vi "HFRR ADV v01.vi"() -> ()   [LabVIEW 2025] (continued)
    "Single" <- "Single - Graph"
  }
  n1798 = disable-structure shown="Disabled" {
    disable-tunnel: [w1922 _] -> w48
    disable-tunnel: _ -> [w1921 _]
    frame Disabled {
      n1799 = while {
        tunnel: w1921 -> [_]
        tunnel: [w1923] -> w1922
        tunnel: [w1924] -> _
        i -> [w1924]
        stop <- w1923 stop-if-true
        w1940 = u16 10 items=["1.0"=10, "1.5"=15, "2.0"=20] ("stop bits (10: 1 bit)")
        n1800 = Wait (ms)(milliseconds to wait=u32 10) -> ()  [unwired: 1 out]
        n1801 = call-poly "VISA Configure Serial Port"("VISA resource name"=refnum<visa-resource-name> "ASRL1::INSTR" ("COM PORT"), "timeout (10sec)"=u32 10, "baud rate (9600)"=u32 57600, "data bits (8)"=u16 8, "stop bits (10: 1 bit)"=w1940) -> ("VISA resource name out"=w1926:refnum<visa-resource-name>, "error out"=w1935:errorcluster)  [unwired: 9 in]
        n1802 = VISA Read(VISA resource name=w1926, byte count=u32 2 ("byte count (0)")) -> (read buffer=w1934:string)  [unwired: 1 in, 3 out]
        n1803 = String Subset(string=w1934, offset (0)=0, length (rest)=2 ("length (rest)")) -> (substring=w1933:string)
        n1804 = Match Pattern(string=w1933, regular expression="<>") -> (offset past match=w1930:i32)  [unwired: 1 in, 3 out]
        n1805 = Greater Or Equal?(x=w1930, y=0) -> (x >= y?=w1925:bool)
        n1806 = case shown="True" w1925 {
          tunnel: w1926 -> [_ w1944]
          tunnel: w1935 -> [_ w1943]
          frame False {
          }
          frame True {
            n1807 = VISA Read(VISA resource name=w1944, byte count=u32 32 ("byte count (0)"), error in (no error)=w1943) -> (read buffer=w1942:string)  [unwired: 3 out]
            n1808 = String Subset(string=w1942, offset (0)=0, length (rest)=8 ("length (rest)")) -> (substring=w1946:string)
            n1809 = String Subset(string=w1942, offset (0)=8, length (rest)=8 ("length (rest)")) -> (substring=w1947:string)
            n1810 = Decimal String To Number(string=w1947) -> (number=w1954:i32)  [unwired: 2 in, 1 out]
            n1811 = Decimal String To Number(string=w1946) -> (number=w1950:i32)  [unwired: 2 in, 1 out]
            n1812 = Divide(x=w1954, y=10000) -> ()  [unwired: 1 out]
            n1813 = Divide(x=w1950, y=1000000) -> ()  [unwired: 1 out]
          }
        }
        n1814 = local read "Quit"() -> (w1923:bool)
      }
    }
    frame Enabled {
    }
  }
  n1815 = Tick Count (ms)() -> (millisecond timer value=w10:u32)
  n1816 = while {
    shift-right: [w2000] -> _
    shift-left: w12 -> [w2004]
    shift-right: [w1999] -> _
    shift-left: w11 -> [w2003]
    shift-right: [w1998] -> _
    shift-left: w12 -> [w2002]
    shift-right: [w1997] -> _
    shift-left: w11 -> [w2001]
    shift-right: [w1995] -> _
    shift-left: w10 -> [w1996]
    shift-right: [w1992] -> _
    shift-left: w9 -> [w1993]
    shift-right: [w1991] -> _
    shift-left: w9 -> [w1994]
    shift-right: [w1984] -> _
    shift-left: w9 -> [w1990]
    shift-right: [w1983] -> _
    shift-left: w9 -> [w1989]
    shift-right: [w1982] -> _
    shift-left: w9 -> [w1988]
    shift-right: [w1981] -> _
    shift-left: w9 -> [w1987]
    shift-right: [w1980] -> _
    shift-left: w9 -> [w1986]
    shift-right: [w1979] -> _
    shift-left: w9 -> [w1985]
    shift-right: [w1978] -> _
    shift-left: w9 -> [w1972]
    shift-right: [w1977] -> _
    shift-left: w9 -> [w1971]
    shift-right: [w1976] -> _
    shift-left: w9 -> [w1970]
    shift-right: [w1975] -> _
    shift-left: w9 -> [w1969]
    shift-right: [w1974] -> _
    shift-left: w9 -> [w1968]
    shift-right: [w1973] -> _
    shift-left: w9 -> [w1967]
    shift-right: [w1958] -> _
    shift-left: w9 -> [w1961]
    shift-right: [w1957] -> _
    shift-left: w9 -> [w1960]
    shift-right: [w1956] -> _
    shift-left: w9 -> [w1959]
    stop <- w2006 stop-if-true
    n1817 = local read "Read UNO"() -> (w1965:string)
    n1818 = local read "Error  2"() -> (w2005:errorcluster)
    n1819 = String Length(string=w1965) -> (length=w1964:i32)
    n1820 = call <vilib>:"Trim Whitespace.vi"("string"=w1965) -> ("trimmed string"=w1966:string)  [unwired: 1 in]
    n1821 = Greater Or Equal?(x=w1964, y=10) -> (x >= y?=w1962:bool)
    n1822 = case shown="No Error" w2005 {
      tunnel: w2004 -> [w2052 w2148]
      tunnel: w2003 -> [w2051 w2147]
      tunnel: w2002 -> [w2050 w2146]
      tunnel: w2001 -> [w2049 w2145]
      tunnel: [w2048 w2148] -> w2000
      tunnel: [w2047 w2147] -> w1999
      tunnel: [w2046 w2146] -> w1998
      tunnel: [w2045 w2145] -> w1997
      tunnel: w1996 -> [w2044 w2144]
      tunnel: [w2043 w2144] -> w1995
      tunnel: w1993 -> [w2042 w2143]
      tunnel: w1994 -> [w2041 w2142]
      tunnel: [w2040 w2143] -> w1992
      tunnel: [w2039 w2142] -> w1991
      tunnel: w1990 -> [w2038 w2141]
      tunnel: w1989 -> [w2037 w2140]
      tunnel: w1988 -> [w2036 w2139]
      tunnel: w1987 -> [w2035 w2138]
      tunnel: w1986 -> [w2034 w2137]
      tunnel: w1985 -> [w2033 w2136]
      tunnel: [w2032 w2141] -> w1984
      tunnel: [w2031 w2140] -> w1983
      tunnel: [w2030 w2139] -> w1982
      tunnel: [w2029 w2138] -> w1981
      tunnel: [w2028 w2137] -> w1980
      tunnel: [w2027 w2136] -> w1979
      tunnel: w1972 -> [w2026 w2135]
      tunnel: [w2025 w2135] -> w1978
      tunnel: [w2024 w2131] -> w1977
      tunnel: [w2023 w2130] -> w1976
      tunnel: [w2022 w2134] -> w1975
      tunnel: [w2021 w2133] -> w1974
      tunnel: [w2020 w2132] -> w1973
      tunnel: w1971 -> [w2019 w2134]
      tunnel: w1970 -> [w2018 w2133]
      tunnel: w1969 -> [w2017 w2132]
      tunnel: w1968 -> [w2016 w2131]
      tunnel: w1967 -> [w2015 w2130]
      tunnel: w1966 -> [w2014 _]
      tunnel: w1962 -> [w2013 _]
      tunnel: w1961 -> [w2012 w2129]
      tunnel: w1960 -> [w2011 w2128]
      tunnel: w1959 -> [w2010 w2127]
      tunnel: [w2009 w2129] -> w1958
      tunnel: [w2008 w2128] -> w1957
      tunnel: [w2007 w2127] -> w1956
      frame No Error {
        n1823 = case shown="True" w2013 {
          tunnel: w2052 -> [w2068 w2120]
          tunnel: w2051 -> [w2067 w2119]
          tunnel: w2050 -> [w2066 w2118]
          tunnel: w2049 -> [w2065 w2117]
          tunnel: [w2068 w2116] -> w2048
          tunnel: [w2067 w2115] -> w2047
          tunnel: [w2066 w2114] -> w2046
          tunnel: [w2065 w2113] -> w2045
          tunnel: w2044 -> [w2064 w2111]
          tunnel: [w2064 w2110] -> w2043
          tunnel: w2042 -> [w2063 w2109]
          tunnel: w2041 -> [w2062 w2108]
          tunnel: [w2063 w2107] -> w2040
          tunnel: [w2062 w2106] -> w2039
          tunnel: w2038 -> [w2061 w2105]
          tunnel: w2037 -> [w2060 w2104]
          tunnel: w2036 -> [w2059 w2103]
          tunnel: w2035 -> [w2058 w2102]
          tunnel: w2034 -> [w2057 w2101]
          tunnel: w2033 -> [w2056 w2100]
          tunnel: [w2061 w2099] -> w2032
          tunnel: [w2060 w2098] -> w2031
          tunnel: [w2059 w2097] -> w2030
          tunnel: [w2058 w2096] -> w2029
          tunnel: [w2057 w2095] -> w2028
          tunnel: [w2056 w2094] -> w2027
          tunnel: w2026 -> [w2074 w2093]
          tunnel: [w2074 w2092] -> w2025
          tunnel: [w2071 w2091] -> w2024
          tunnel: [w2070 w2090] -> w2023
          tunnel: [w2073 w2089] -> w2022
          tunnel: [w2069 w2088] -> w2021
          tunnel: [w2072 w2087] -> w2020
          tunnel: w2019 -> [w2073 w2086]
          tunnel: w2018 -> [w2072 w2085]
          tunnel: w2017 -> [w2071 w2084]
          tunnel: w2016 -> [w2070 w2083]
          tunnel: w2015 -> [w2069 w2082]
          tunnel: w2014 -> [_ w2081]
          tunnel: w2012 -> [w2055 w2080]
          tunnel: w2011 -> [w2054 w2079]
          tunnel: w2010 -> [w2053 w2078]
          tunnel: [w2055 w2077] -> w2009
          tunnel: [w2054 w2076] -> w2008
          tunnel: [w2053 w2075] -> w2007
          frame False {
          }
          frame True {
            n1824 = Tick Count (ms)() -> (millisecond timer value=w2112:u32)
            n1825 = String To Byte Array(string=w2081) -> (unsigned byte array=w2125:u8[])
            n1826 = Array Size(array=w2125) -> (size(s)=w2124:i32)
            n1827 = formula code="// --- INTERNAL VARIABLE DECLARATIONS ---\nint i = 0;\nint k = 0;\nint start_idx = 0;\nint end_idx = 0;\nint phase = 0;\nint ch0_val = 0;    \nint ch1_val = 0;    \nfloat ch0_raw = 0.0;\nfloat ch1_raw = 0.0;\nfloat temp0 = 0.0;\nfloat temp1 = 0.0;\nfloat ch0_clean = 0.0;\nfloat ch1_clean = 0.0;\n\nint valid_samples = 0; // Track if we actually parsed new data this window\nfloat max_allowed_bits = 8388607.0; // ADC max value\n\n// Temporal intermediate variables for calculation smoothing\nfloat raw_p2p_v = 0.0;\nfloat raw_friction = 0.0;\nfloat raw_cof = 0.0;\n\n// Temporal intermediate variables for Piezo voltage translations\nfloat piezo_min_v = 0.0;\nfloat piezo_max_v = 0.0;\n\n// Initialize output variables to current shift register states right away\nout_LVDT_Min_V = in_LVDT_Min_V;\nout_LVDT_Max_V = in_LVDT_Max_V;\nout_LVDT_P2P_V = in_LVDT_P2P_V;\nout_Piezo_P2P = in_Piezo_P2P;\nout_Friction_N = in_Friction_N;\nout_COF = in_COF;\nwindow_ready = 0;\n\n// --- STEP 1: PARSE EVERY STRING IN THE BYTE ARRAY (UPDATED FOR CH1;CH2) ---\nif (array_size > 0) {\n    ch0_val = 0;\n    ch1_val = 0;\n    phase = 0;\n    int has_digits = 0;\n\n    for (i = 0; i < array_size; i++) {\n        // Skip newline or CR carriage returns if present\n        if (raw_bytes[i] == 10 || raw_bytes[i] == 13) {\n            continue;\n        }\n\n        if (raw_bytes[i] == 59) { // ';' delimiter switches to CH2\n            phase = 1;\n        } \n        else if (raw_bytes[i] >= 48 && raw_bytes[i] <= 57) { // ASCII digits '0'-'9'\n            has_digits = 1;\n            if (phase == 0) {\n                ch0_val = (ch0_val * 10) + (raw_bytes[i] - 48);\n            } else {\n                ch1_val = (ch1_val * 10) + (raw_bytes[i] - 48);\n            }\n        }\n    }\n\n    // Only process if both channels were parsed successfully\n    if (phase == 1 && has_digits) {\n        ch0_raw = ch0_val * 1.0;\n        ch1_raw = ch1_val * 1.0;\n\n        // Hard-clamping to catch sudden massive ASCII noise spikes\n        if (ch0_raw > max_allowed_bits)  ch0_raw = max_allowed_bits;\n        if (ch0_raw < -max_allowed_bits) ch0_raw = -max_allowed_bits;\n        if (ch1_raw > max_allowed_bits)  ch1_raw = max_allowed_bits;\n        if (ch1_raw < -max_allowed_bits) ch1_raw = -max_allowed_bits;\n\n        // --- STEP 2: 3-SAMPLE MEDIAN FILTER ---\n        m0_2 = m0_1; m0_1 = m0_0; m0_0 = ch0_raw;\n        float s0_0 = m0_0; float s0_1 = m0_1; float s0_2 = m0_2;\n        if (s0_0 > s0_1) { temp0 = s0_0; s0_0 = s0_1; s0_1 = temp0; }\n        if (s0_1 > s0_2) { temp0 = s0_1; s0_1 = s0_2; s0_2 = temp0; }\n        if (s0_0 > s0_1) { temp0 = s0_0; s0_0 = s0_1; s0_1 = temp0; }\n        ch0_clean = s0_1;\n\n        m1_2 = m1_1; m1_1 = m1_0; m1_0 = ch1_raw;\n        float s1_0 = m1_0; float s1_1 = m1_1; float s1_2 = m1_2;\n        if (s1_0 > s1_1) { temp1 = s1_0; s1_0 = s1_1; s1_1 = temp1; }\n        if (s1_1 > s1_2) { temp1 = s1_1; s1_1 = s1_2; s1_2 = temp1; }\n        if (s1_0 > s1_1) { temp1 = s1_0; s1_0 = s1_1; s1_1 = temp1; }\n        ch1_clean = s1_1;\n\n        // --- STEP 3: EXPONENTIAL FILTER (STREAM LEVEL) ---\n        if (ch0_filt == 0.0) ch0_filt = ch0_clean;\n        if (ch1_filt == 0.0) ch1_filt = ch1_clean;\n\n        ch0_filt = ch0_filt + (ch0_clean - ch0_filt) * 0.125;\n        ch1_filt = ch1_filt + (ch1_clean - ch1_filt) * 0.125;\n\n        // --- STEP 4: MIN/MAX WINDOW CONTINUOUS ACCUMULATION ---\n        if (ch0_filt > max_ch0) max_ch0 = ch0_filt;\n        if (ch0_filt < min_ch0) min_ch0 = ch0_filt;\n        if (ch1_filt > max_ch1) max_ch1 = ch1_filt;\n        if (ch1_filt < min_ch1) min_ch1 = ch1_filt;\n\n        valid_samples++; // Successfully parsed and accumulated a clean point\n    }\n}\n\n// --- STEP 5: WINDOW EVALUATION ENGINE ---\nif (((current_time_ms - start_time_ms) >= 50) && (valid_samples > 0) && (min_ch0 < 9000000.0) && (min_ch1 < 9000000.0)) {\n    window_ready = 1;\n\n    // Linear Bit-to-Voltage Transformations (LVDT - Channel 0)\n    out_LVDT_Min_V = (min_ch0 * VREF) / 8388607.0;\n    out_LVDT_Max_V = (max_ch0 * VREF) / 8388607.0;\n    raw_p2p_v = out_LVDT_Max_V - out_LVDT_Min_V;\n\n    // Linear Bit-to-Voltage Transformations (Piezo - Channel 1)\n    piezo_min_v = (min_ch1 * VREF) / 8388607.0;\n    piezo_max_v = (max_ch1 * VREF) / 8388607.0;\n    \n    // Assign Peak-to-Peak Voltage directly to output indicator\n    out_Piezo_P2P = piezo_max_v - piezo_min_v;\n    \n    // Force scaling calculations using Voltage delta * Newtons/Volt Factor\n    raw_friction = out_Piezo_P2P * PIEZO_CAL_FACTOR ;\n    raw_cof = raw_friction / NORMAL_FORCE;\n\n    // --- STEP 6: OUTPUT METRIC SMOOTHING (Low-Pass Filter Alpha = 0.05) ---\n    // Seed initial historical metrics if first loop iteration\n    if (hist_LVDT_P2P == 0.0) hist_LVDT_P2P = raw_p2p_v;\n    if (hist_Friction == 0.0) hist_Friction = raw_friction;\n    if (hist_COF == 0.0)      hist_COF = raw_cof;\n\n    // Apply exponential output dampening\n    hist_LVDT_P2P = hist_LVDT_P2P + (raw_p2p_v - hist_LVDT_P2P) * 0.05;\n    hist_Friction = hist_Friction + (raw_friction - hist_Friction) * 0.05;\n    hist_COF      = hist_COF + (raw_cof - hist_COF) * 0.05;\n\n    // Direct smoothed parameters out to UI Indicators\n    out_LVDT_P2P_V = hist_LVDT_P2P;\n    out_Friction_N = hist_Friction;\n    out_COF        = hist_COF;\n\n    // Reset tracking targets to extreme boundaries safely\n    min_ch0 = 9999999.0;\n    max_ch0 = -9999999.0;\n    min_ch1 = 9999999.0;\n    max_ch1 = -9999999.0;\n\n    valid_samples = 0; // Reset counter for next time frame\n    start_time_ms = current_time_ms;\n}"("raw_bytes"=w2125, "array_size"=w2124, "VREF"="VREF", "PIEZO_CAL_FACTOR"="PIEZO_CAL_FACTOR", "NORMAL_FORCE"="NORMAL_FORCE", "min_ch0"=w2120, "max_ch0"=w2119, "min_ch1"=w2118, "max_ch1"=w2117, "current_time_ms"=w2112, "start_time_ms"=w2111, "ch0_filt"=w2109, "ch1_filt"=w2108, "m0_0"=w2105, "m0_1"=w2104, "m0_2"=w2103, "m1_0"=w2102, "m1_1"=w2101, "m1_2"=w2100, "in_LVDT_Min_V"=w2093, "in_LVDT_Max_V"=w2086, "in_LVDT_P2P_V"=w2085, "in_Piezo_P2P"=w2084, "in_Friction_N"=w2083, "in_COF"=w2082, "hist_LVDT_P2P"=w2080, "hist_Friction"=w2079, "hist_COF"=w2078) -> ("window_ready"=→"Valid_data":dbl, "out_LVDT_Min_V"=w2092:dbl, "out_LVDT_Max_V"=w2091:dbl, "out_LVDT_P2P_V"=w2090:dbl, "out_Piezo_P2P"=w2089:dbl, "out_Friction_N"=w2088:dbl, "out_COF"=w2087:dbl, "min_ch0"=w2116:dbl, "max_ch0"=w2115:dbl, "min_ch1"=w2114:dbl, "max_ch1"=w2113:dbl, "start_time_ms"=w2110:u32, "ch0_filt"=w2107:dbl, "ch1_filt"=w2106:dbl, "m0_0"=w2099:dbl, "m0_1"=w2098:dbl, "m0_2"=w2097:dbl, "m1_0"=w2096:dbl, "m1_1"=w2095:dbl, "m1_2"=w2094:dbl, "hist_LVDT_P2P"=w2077:dbl, "hist_Friction"=w2076:dbl, "hist_COF"=w2075:dbl)
            "LVDT MIN" <- w2092
            "LVDT MAX" <- w2091
            "LVDT Peak" <- w2090
            "pizo raw" <- w2089
            "cof" <- w2087
            "Frictioin Force Raw" <- w2088
          }
        }
      }
      frame Error {
      }
    }
    n1828 = local read "Quit"() -> (w2006:bool)
  }
  n1829 = disable-structure shown="Disabled" {
    disable-tunnel: errorcluster {"status"=TRUE, "code"=0, "source"="Init"} ("error IO") -> [w2151 _]
    disable-tunnel: [w2149 _] -> w51
    frame Disabled {
      n1830 = while {
        shift-right: [w2167] -> w2153
        shift-left: _ -> [w2158]
        shift-right: [w2166] -> w2152
        shift-left: w2151 -> [w2160]
        tunnel: [w2155] -> w2149
        tunnel: [w2165] -> _
        i -> [w2165]
        stop <- w2155 stop-if-true
        n1831 = local read "Port 1a"() -> (w2161:bool)
        n1832 = local read "Port 3"() -> (w2162:bool)
        n1833 = local read "Com Port 1"() -> (w2159:refnum<visa-resource-name>)
        n1834 = Or(x=w2162, y=w2161) -> (x .or. y?=w2164:bool)
        n1835 = Unbundle(w2160) -> ("status"=→"Port 3":bool)  [unwired: 2 out]
        n1836 = Not Equal?(x=w2159, y=w2158) -> (x != y?=w2156:bool)
        n1837 = case shown="True" w2164 {
          frame False {
            w2170 = TRUE ("Visible")
            n1838 = property on="Port 1a" class="Bool (strict)"("Visible"=w2170) -> ()  [unwired: 2 in, 2 out]
            n1839 = property on="Port 3" class="Bool (strict)"("Visible"=w2170) -> ()  [unwired: 2 in, 2 out]
          }
          frame True {
            w2171 = TRUE ("Visible")
            n1840 = property on="Port 1a" class="Bool (strict)"("Visible"=w2171) -> ()  [unwired: 2 in, 2 out]
            n1841 = property on="Port 3" class="Bool (strict)"("Visible"=w2171) -> ()  [unwired: 2 in, 2 out]
          }
        }
        n1842 = Wait (ms)(milliseconds to wait=u32 40) -> ()  [unwired: 1 out]
        n1843 = case shown="True" w2156 {
          tunnel: [w2168 errorcluster {"status"=TRUE, "code"=0, "source"="Init"} ("error out")] -> w2157
          tunnel: w2160 -> [w2168 _]
          frame False {
          }
          frame True {
          }
        }
        n1844 = case shown="Error" w2157 {
          selector: w2157 -> [w2178 w2196]
          tunnel: [w2181 w2200] -> w2167
          tunnel: [w2180 w2194] -> w2166
          tunnel: w2158 -> [w2179 w2198]
          frame No Error {
            n1845 = property class="Instr"(reference=w2179, error in=w2178) -> (reference out=w2176:refnum<visa-resource-name>, error out=w2177:errorcluster, "Serial Settings:Number of Bytes at Serial Port"=w2173:u32)
            n1846 = Greater?(x=w2173, y=u32 5) -> (0:w2172:bool)
            n1847 = Not(x=w2172) -> (.not. x?=→"Port 1a":bool)
            n1848 = while {
              tunnel: [w2189] -> w2180
              tunnel: [w2188] -> w2181
              tunnel: w2177 -> [w2187]
              tunnel: w2176 -> [w2186]
              stop <- TRUE stop-if-true
              n1849 = property class="Instr" props=["Serial Settings:Number of Bytes at Serial Port"](reference=w2186, error in=w2187) -> (reference out=w2191:refnum<visa-resource-name>, error out=w2190:errorcluster)  [unwired: 1 out]
              n1850 = VISA Read(VISA resource name=w2191, byte count=u32 50, error in (no error)=w2190) -> (VISA resource name out=w2188:refnum<visa-resource-name>, read buffer=w2183:string, error out=w2189:errorcluster)  [unwired: 1 out]
              n1851 = Wait (ms)(milliseconds to wait=u32 5) -> ()  [unwired: 1 out]
            }
          }
          frame Error {
            w2206 = u16 0 items=["None", "XON/XOFF", "RTS/CTS", "XON/XOFF & RTS/CTS", "DTR/DSR", "XON/XOFF & DTR/DSR"] ("flow control (0:none)  2")
            w2204 = u16 10 items=["1.0"=10, "1.5"=15, "2.0"=20] ("stop bits 2")
            w2202 = u16 0 items=["None", "Odd", "Even", "Mark", "Space"] ("parity 2")
            w2203 = u32 10000  # timeout (10sec)
            n1852 = VISA Close(VISA resource name=w2198, error in (no error)=w2196) -> (error out=w2199:errorcluster)
            n1853 = local write "Port 1a"(FALSE ("Port 1a")) -> ()
            n1854 = local read "Com Port 1"() -> (w2193:refnum<visa-resource-name>)
            n1855 = call <vilib>:"Clear Errors.vi"("error in (no error)"=w2199) -> ("error out"=w2197:errorcluster)  [unwired: 5 in, 1 out]
            n1856 = call-poly "VISA Configure Serial Port"("VISA resource name"=w2193, "timeout (10sec)"=w2203, "baud rate (9600)"=u32 250000 ("baud rate  2"), "data bits (8)"=u16 8 ("data bits  2"), "parity (0:none)"=w2202, "error in (no error)"=w2197, "stop bits (10: 1 bit)"=w2204, "flow control (0:none)"=w2206) -> ("VISA resource name out"=w2207:refnum<visa-resource-name>, "error out"=w2208:errorcluster)  [unwired: 6 in]
            n1857 = flat-sequence {
              tunnel: w2207 -> [w2210]
              tunnel: w2208 -> [w2209]
              tunnel: [w2210] -> w2200
              tunnel: [w2209] -> w2194
              frame #0 {
                n1858 = Wait (ms)(milliseconds to wait=u32 50) -> ()  [unwired: 1 out]
              }
            }
            "Residual Uno" <- ""
          }
        }
        n1859 = local read "Quit"() -> (w2155:bool)
        "Error Uno" <- w2160
      }
      n1860 = VISA Close(VISA resource name=w2153, error in (no error)=w2152) -> (error out=w2150:errorcluster)
      n1861 = call <vilib>:"Clear Errors.vi"("error in (no error)"=w2150) -> ()  [unwired: 5 in, 2 out]
    }
    frame Enabled {
    }
  }
  n1862 = while {
    stop <- w2221 stop-if-true
    # "V0OLTAGE TO STROKE (peice vise calibration)"
    n1863 = local read "LVDT MIN"() -> (w2213:dbl)
    n1864 = local read "LVDT Peak"() -> (w2212:dbl)
    n1865 = Wait (ms)(milliseconds to wait=u32 10) -> ()  [unwired: 1 out]
    n1866 = formula code="// Dynamic Parameterized Linear Interpolation Node\n// Inputs: vpp_val, voltages (Array), distances (Array)\n// Outputs: stroke\n\nint i = 0;\nint segments = 11; // 12 points make 11 interpolation segments\n\n// 1. Lower Boundary Clamp\nif (vpp_val <= voltages[0]) {\n    stroke = distances[0];\n}\n// 2. Upper Boundary Clamp\nelse if (vpp_val >= voltages[segments]) {\n    stroke = distances[segments];\n}\n// 3. Dynamic Segment Search Loop\nelse {\n    stroke = distances[0]; // Fallback baseline\n    for (i = 0; i < segments; i++) {\n        if (vpp_val >= voltages[i] && vpp_val <= voltages[i+1]) {\n            // Standard linear interpolation formula using array lookups\n            stroke = distances[i] + (vpp_val - voltages[i]) * (distances[i+1] - distances[i]) / (voltages[i+1] - voltages[i]);\n            break; // Segment found, safely exit the loop\n        }\n    }\n}"("vpp_val"=w2212, "voltages"="calibration values", "distances"="STROKE") -> ("stroke"=→"LVDT STROKE":dbl)
    n1867 = local read "Calibration Tare Value"() -> (w2217:dbl)
    n1868 = local read "Calibration Tare"() -> (w2215:bool)
    n1869 = Subtract(x=w2213, y=w2217) -> (x-y=→"LVDT STROKE  Calibration":dbl)
    n1870 = case shown="True" w2215 {
      selector: w2215 -> [_ w2223]
      tunnel: w2213 -> [_ w2224]
      frame False {
      }
      frame True {
        n1871 = Not(x=w2223) -> (.not. x?=w2222:bool)
        n1872 = local write "Calibration Tare"(w2222) -> ()
        "Calibration Tare Value" <- w2224
      }
    }
    n1873 = local read "Quit"() -> (w2221:bool)
  }
  n1874 = while {
    stop <- w2247 stop-if-true
    n1875 = local read "Due read"() -> (w2245:string)
    n1876 = call <vilib>:"High Resolution Polling Wait.vi"("seconds to wait"=0.02) -> ()  [unwired: 10 in, 1 out]
    n1877 = local read "Frictioin Force Raw"() -> (w2227:dbl)
    n1878 = Spreadsheet String To Array(delimiter (Tab)=";", format string="", spreadsheet string=w2245, array type (2D Dbl)=string[] []) -> (array=w2242:string[])
    n1879 = Fract/Exp String To Number(string=w2242) -> (number=w2241:dbl[])  [unwired: 3 in, 1 out]
    n1880 = call <vilib>:"Median Filter PtByPt.vi"("rank"=2, "x"=w2227) -> ("Filtered x"=→"Friction":dbl)  [unwired: 2 in, 1 out]
    n1881 = Index Array(array=w2241) -> (element #1=→"Sample Temperature 2":dbl, element #2=→"Target Sample Temperature":dbl, element #3=→"Current Duty Cycle":dbl, element #4=→"Ambient Temperature":dbl, element #5=→"Dac Status":dbl, element #6=→"Vpp":dbl, element #7=→"Active Error Code":dbl, element #8=→"Kp":dbl, element #9=→"Ki":dbl, element #10=→"Kd":dbl, element #11=→"SampleRaw":dbl, element #12=→"AmbRaw":dbl)  [unwired: 12 in]
    n1882 = local read "Quit"() -> (w2247:bool)
  }
  n1883 = while {
    shift-right: [w2261] -> w47
    shift-left: _ -> [w2253]
    shift-right: [w2248] -> w46
    shift-left: errorcluster {"status"=FALSE, "code"=0, "source"="Init"} ("error out") -> [w2255]
    tunnel: [w2250] -> w50
    tunnel: [w2260] -> _
    i -> [w2260]
    stop <- w2250 stop-if-true
    n1884 = local read "Com Port 2"() -> (w2254:refnum<visa-resource-name>)
    n1885 = local read "Port 2a"() -> (w2256:bool)
    n1886 = Unbundle(w2255) -> ("status"=→"Port 4":bool)  [unwired: 2 out]
    n1887 = call <vilib>:"High Resolution Polling Wait.vi"("seconds to wait"=0.02) -> ()  [unwired: 10 in, 1 out]
    n1888 = local read "Port 4"() -> (w2257:bool)
    n1889 = Not Equal?(x=w2254, y=w2253) -> (x != y?=w2252:bool)
    n1890 = Or(x=w2257, y=w2256) -> (x .or. y?=w2259:bool)
    n1891 = case shown="False" w2259 {
      frame False {
        w2264 = TRUE ("Visible")
        n1892 = property on="Port 2a" class="Bool (strict)"("Visible"=w2264) -> ()  [unwired: 2 in, 2 out]
        n1893 = property on="Port 4" class="Bool (strict)"("Visible"=w2264) -> ()  [unwired: 2 in, 2 out]
      }
      frame True {
        w2265 = TRUE ("Visible")
        n1894 = property on="Port 2a" class="Bool (strict)"("Visible"=w2265) -> ()  [unwired: 2 in, 2 out]
        n1895 = property on="Port 4" class="Bool (strict)"("Visible"=w2265) -> ()  [unwired: 2 in, 2 out]
      }
    }
    n1896 = case shown="True" w2252 {
      tunnel: [w2262 errorcluster {"status"=TRUE, "code"=0, "source"="Init"} ("error out")] -> w2251
      tunnel: w2255 -> [w2262 _]
      frame False {
      }
      frame True {
      }
    }
    n1897 = case shown="No Error" w2251 {
      selector: w2251 -> [w2278 w2309]
      tunnel: [w2271 w2314] -> w2261
      tunnel: [w2279 w2307] -> w2248
      tunnel: w2253 -> [w2280 w2312]
      frame No Error {
        n1898 = property class="Instr" props=["Serial Settings:Number of Bytes at Serial Port"](reference=w2280, error in=w2278) -> (reference out=w2272:refnum<visa-resource-name>, error out=w2277:errorcluster)  [unwired: 1 out]
        n1899 = while {
          tunnel: [w2288] -> w2273
          tunnel: [w2287] -> w2274
          tunnel: w2277 -> [w2286]
          tunnel: w2272 -> [w2285]
          tunnel: [w2284] -> _
          i -> [w2284]
          stop <- TRUE stop-if-true
          n1900 = property class="Instr" props=["Serial Settings:Number of Bytes at Serial Port"](reference=w2285, error in=w2286) -> (reference out=w2290:refnum<visa-resource-name>, error out=w2289:errorcluster)  [unwired: 1 out]
          n1901 = VISA Read(VISA resource name=w2290, byte count=u32 1000, error in (no error)=w2289) -> (VISA resource name out=w2287:refnum<visa-resource-name>, read buffer=→"Due read":string, error out=w2288:errorcluster)  [unwired: 1 out]
        }
        n1902 = local read "Due Write"() -> (w2270:string)
        n1903 = call <vilib>:"Trim Whitespace.vi"("string"=w2270) -> ("trimmed string"=w2269:string)  [unwired: 1 in]
        n1904 = Not Equal?(x=w2269, y="") -> (x != y?=w2275:bool)
        n1905 = VISA Flush I/O Buffer(VISA resource name=w2274) -> (VISA resource name out=w2267:refnum<visa-resource-name>, error out=→"error out 10":errorcluster)  [unwired: 2 in]
        n1906 = case shown="True" w2275 {
          tunnel: w2267 -> [w2292 w2297]
          tunnel: [w2292 w2301] -> w2271
          tunnel: w2273 -> [w2291 w2296]
          tunnel: [w2291 w2299] -> w2279
          tunnel: w2269 -> [_ w2295]
          tunnel: [_ w2298] -> _
          frame False {
            # "DATA  WRITE LOOP"
          }
          frame True {
            n1907 = Concatenate Strings(w2295, "\r\n") -> (w2294:string)
            n1908 = VISA Write(VISA resource name=w2297, write buffer=w2294, error in (no error)=w2296) -> (VISA resource name out=w2301:refnum<visa-resource-name>, return count=w2298:u32, error out=w2300:errorcluster)
            n1909 = flat-sequence {
              tunnel: w2300 -> [w2303]
              tunnel: [w2303] -> w2299
              frame #0 {
                n1910 = local write "Due Write"("" ("Command")) -> ()
                n1911 = Wait (ms)(milliseconds to wait=u32 5) -> ()  [unwired: 1 out]
              }
            }
          }
        }
        "Port 2a" <- TRUE ("Port 2a")
      }
      frame Error {
        w2320 = u16 0 items=["None", "XON/XOFF", "RTS/CTS", "XON/XOFF & RTS/CTS", "DTR/DSR", "XON/XOFF & DTR/DSR"] ("flow control (0:none)  2")
        w2318 = u16 10 items=["1.0"=10, "1.5"=15, "2.0"=20] ("stop bits 2")
        w2316 = u16 0 items=["None", "Odd", "Even", "Mark", "Space"] ("parity 2")
        w2317 = u32 10000  # timeout (10sec)
        n1912 = VISA Clear(VISA resource name=w2312, error in (no error)=w2309) -> (VISA resource name out=w2311:refnum<visa-resource-name>, error out=w2310:errorcluster)
        n1913 = VISA Close(VISA resource name=w2311, error in (no error)=w2310) -> (error out=w2313:errorcluster)
        n1914 = call <vilib>:"Clear Errors.vi"("error in (no error)"=w2313) -> ()  [unwired: 5 in, 2 out]
        n1915 = local write "Port 2a"(FALSE ("Port 2a")) -> ()
        n1916 = local read "Com Port 2"() -> (w2306:refnum<visa-resource-name>)
        "visa due" <- w2306
        n1917 = call-poly "VISA Configure Serial Port"("VISA resource name"=w2306, "timeout (10sec)"=w2317, "baud rate (9600)"=u32 250000 ("baud rate  2"), "data bits (8)"=u16 8 ("data bits  2"), "parity (0:none)"=w2316, "stop bits (10: 1 bit)"=w2318, "flow control (0:none)"=w2320) -> ("VISA resource name out"=w2321:refnum<visa-resource-name>, "error out"=w2322:errorcluster)  [unwired: 7 in]
        n1918 = flat-sequence {
          tunnel: w2321 -> [w2324]
          tunnel: w2322 -> [w2323]
          tunnel: [w2324] -> w2314
          tunnel: [w2323] -> w2307
          frame #0 {
            n1919 = Wait (ms)(milliseconds to wait=u32 50) -> ()  [unwired: 1 out]
          }
        }
        "Residual Due" <- ""
      }
    }
    "error out 9" <- w2248
    n1920 = local read "Quit"() -> (w2250:bool)
    "Error Due" <- w2255
  }
  n1921 = local write "FRICVALZ"(0.0 ("FRICVALZ")) -> ()
  n1922 = while {
    tunnel: [w2328] -> _
    tunnel: [w2327] -> w60
    i -> [w2328]
    stop <- w2327 stop-if-true
    n1923 = property on="DEMO" class="Bool (strict)"() -> ("Value"=w2326:bool)  [unwired: 2 in, 2 out]
    n1924 = case shown="True" w2326 {
      frame False {
        n1925 = local read "conststatus"() -> (w2333:dbl)
        n1926 = local read "Main Tab"() -> (w2331:T4)
        n1927 = local read "EDIT"() -> (w2346:bool)
        n1928 = local read "Rate"() -> (w2345:dbl)
        n1929 = case shown="True" w2346 {
          tunnel: [FALSE TRUE] -> _
          frame False {
          }
          frame True {
          }
        }
        n1930 = Equal?(x=w2331, y=T29."About" ("Main Tab")) -> (x = y?=w2339:bool)
        n1931 = Wait (ms)(milliseconds to wait=u32 50) -> ()  [unwired: 1 out]
        n1932 = Equal?(x=w2333, y=0.0) -> (x = y?=w2334:bool)
        n1933 = Divide(x=1.0, y=w2345) -> (x/y=w2341:dbl)
        "Time 2" <- w2341
        n1934 = case shown="True" w2334 {
          frame False {
          }
          frame True {
            # "C:\\WinDucom\\calibrate WO 2391.dcf"
            n1935 = local write "Lan flag"(22) -> ()
            n1936 = local write "conststatus"(10.0 ("rpm value : 2")) -> ()
            n1937 = String To Path(string="C:\\LAB-IQ\\calibrate WO 2472.dcf") -> (path=w2352:path)
            n1938 = Open/Create/Replace File "Open File"(file path (use dialog)=w2352) -> (refnum out=w2350:refnum<file>)  [unwired: 5 in, 2 out]
            n1939 = for {
              N: 23 -> [_]
              tunnel: w2350 -> [w2361]
              i -> [w2355]
              (unwired) TRUE ("line mode (F)")
              n1940 = Read from Text File "Read File"(file (use dialog)=w2361) -> (text=w2360:string)  [unwired: 3 in, 3 out]
              n1941 = Match Pattern(string=w2360, regular expression="]") -> (after substring=w2358:string)  [unwired: 1 in, 3 out]
              n1942 = String Subset(string=w2360, offset (0)=5, length (rest)=10 ("length (rest)")) -> (substring=w2353:string)
              n1943 = Fract/Exp String To Number(string=w2353) -> (number=w2354:dbl)  [unwired: 3 in, 1 out]
              n1944 = Match Pattern(string=w2358, regular expression="-") -> (before substring=w2356:string)  [unwired: 1 in, 3 out]
              n1945 = case shown="10" w2355 {
                tunnel: w2354 -> [_ _ _ _ _ _ _ _ _ _ w2368 _ _ _ _ _ _ _ _ _ _ _ _ _]
                tunnel: w2356 -> [_ _ _ _ w2364 w2365 w2366 _ _ _ _ _ _ _ _ _ _ _ _ _ w2369 w2370 w2371 _]
                frame 0 {
                }
                frame 1 {
                }
                frame 2 {
                }
                frame 3 {
                }
                frame 4 {
                  n1946 = local write "Com Port 1"(w2364) -> ()
                }
                frame 5 {
                  n1947 = local write "Com Port 2"(w2365) -> ()
                  n1948 = local write "visa due"(w2365) -> ()
                }
                frame 6 {
                  n1949 = String To Path(string=w2366) -> (path=w2367:path)
                  n1950 = local write "File Path"(w2367) -> ()
                  "String" <- w2366
                }
                frame 7 {
                }
                frame 8 {
                }
                frame 9 {
                }
                frame 10 {
                  n1951 = local write "Language Selection"(w2368) -> ()
                }
                frame 11 {
                }
                frame 12 {
                }
                frame 13 {
                }
                frame 14 {
                }
                frame 15 {
                }
                frame 16 {
                }
                frame 17 {
                }
                frame 18 {
                }
                frame 21 {
                }
                frame 22 {
                  n1952 = local write "Com Port 3"(w2369) -> ()
                }
                frame 20 {
                  n1953 = local write "Camera Port :"(w2370) -> ()
                }
                frame 19 {
                  n1954 = local write "C3 :"(w2371) -> ()
                }
                frame 23, Default {
                }
              }
            }
          }
        }
        n1955 = Select(t=u32 2500 ("milliseconds to wait"), s=w2339, f=u32 500 ("milliseconds to wait")) -> (s? t:f=w2337:u32)
        n1956 = Multiply(x=w2341, y=w2337) -> (x*y=w2343:dbl)
        n1957 = call "Elapsed Time2"("Time Target (s)"=w2343, "Auto Reset"=TRUE) -> ("Time has Elapsed"=w2335:bool)  [unwired: 10 in, 7 out]
        n1958 = case shown="True" w2335 {
          frame False {
          }
          frame True {
            n1959 = stacked-sequence {
              frame #0 {
                # "DATA PROCESSING"
                # "115 mV/N"
                n1960 = local read "Sample Temperature 2"() -> (w2374:dbl)
                n1961 = local read "RH Numeric:"() -> (→"Humidity ( %RH )":dbl)
                n1962 = local read "FRICVALZ"() -> (w2391:dbl)
                n1963 = local read "Friction"() -> (w2377:dbl)
                n1964 = call <vilib>:"Mean PtByPt.vi"("x"=w2374, "sample length"=100) -> ("mean"=w2373:dbl)  [unwired: 2 in, 1 out]
                "TEMP 2" <- w2373
                "TEMP 3" <- w2373
                n1965 = Subtract(x=w2377, y=w2391) -> (x-y=w2386:dbl)
                "FF 2" <- w2386
                "FF 4" <- w2386
                n1966 = local read "Ambient Temperature"() -> (→"AIR TEMP":dbl)
                n1967 = local read "TEMP"() -> (w2390:dbl)
                n1968 = local write "FF 3"(w2386) -> ()
                n1969 = Compound Arithmetic op=OR("FRICVALZ 4", "FRICVALZ 3", "FRICVALZ 2") -> (w2382:bool)
                n1970 = case shown="True" w2382 {
                  tunnel: w2377 -> [_ w2397]
                  frame False {
                  }
                  frame True {
                    w2396 = FALSE ("FRICVALZ")
                    n1971 = local write "FRICVALZ 3"(w2396) -> ()
                    n1972 = local write "FRICVALZ 2"(w2396) -> ()
                    n1973 = local write "FRICVALZ 4"(w2396) -> ()
                    "FRICVALZ" <- w2397
                  }
                }
                n1974 = Not A Number/Path/Refnum?(number/path/refnum=w2390) -> (NaN/Path/Refnum?=w2389:bool)
                n1975 = Not A Number/Path/Refnum?(number/path/refnum=w2386) -> (NaN/Path/Refnum?=w2388:bool)
                n1976 = Divide(x=w2386, y=1.96) -> (x/y=w2383:dbl)
                n1977 = Compound Arithmetic op=OR(w2389, w2388) -> (w2387:bool)
                n1978 = Not A Number/Path/Refnum?(number/path/refnum=w2383) -> (NaN/Path/Refnum?=w2384:bool)
                n1979 = case shown="True" w2387 {
                  frame False {
                  }
                  frame True {
                    n1980 = local write "TEMP"(0.0 ("TEMP")) -> ()
                    n1981 = local write "FF 2"(0.0 ("FF 2")) -> ()
                    n1982 = local write "reinit"(TRUE ("reinit")) -> ()
                  }
                }
                n1983 = local write "TEMP"(w2373) -> ()
                n1984 = Select(t=0.0, s=w2384, f=w2383) -> (s? t:f=w2376:dbl)
                "COF 2" <- w2376
                n1985 = local write "COF 3"(w2376) -> ()
              }
            }
          }
        }
        "Rate" <- 2500.0 ("No of Samples")
      }
      frame True {
        n1986 = Wait (ms)(milliseconds to wait=u32 500) -> ()  [unwired: 1 out]
      }
    }
    n1987 = local read "Quit"() -> (w2327:bool)
  }
  n1988 = property on="RUN" class="Bool (strict)"("Visible"=TRUE) -> ()  [unwired: 2 in, 2 out]
  n1989 = while {
    tunnel: [w2418] -> _
    tunnel: [w2401] -> w62
    tunnel: w7 -> [_]
    i -> [w2418]
    stop <- w2401 stop-if-true
    # "C:\\LAB-IQ-NXT\\Scar View.exe"
    n1990 = local read "OK Button 16"() -> (w2408:bool)
    n1991 = local read "Main Tab"() -> (w2402:T4)
    n1992 = local read "service 3"() -> (w2403:bool)
    n1993 = local read "OPEN 6"() -> (w2405:bool)
    n1994 = local read "EDIT 2"() -> (w2407:bool)
    n1995 = flat-sequence {
      frame #0 {
        n1996 = stacked-sequence {
          frame #0 {
            n1997 = local read "EDIT"() -> (w2896:bool)
            n1998 = case shown="False" w2896 {
              tunnel: [u8 2 ("Disabled") u8 0 ("Disabled")] -> _
              frame False {
                w2898 = FALSE
                n1999 = local write "Password"("") -> ()
                n2000 = local write "x = y?"(w2898) -> ()
                n2001 = property on="Password" class="Str"("Visible"=w2898) -> ()  [unwired: 2 in, 2 out]
              }
              frame True {
                n2002 = property on="Password" class="Str"("Visible"=TRUE) -> ()  [unwired: 2 in, 2 out]
              }
            }
            "dipl pwd" <- "@143$\n" ("dipl pwd")
          }
          frame #1 {
          }
          frame #2 {
          }
          frame #3 {
          }
          frame #4 {
            n2003 = String To Byte Array(string="Password") -> (unsigned byte array=w2909:u8[])
            n2004 = Search 1D Array(1D array=w2909, element=u8 10) -> (index of element=w2907:i32)  [unwired: 1 in]
            n2005 = Index Array(array=w2909, index=w2907) -> (element=w2908:u8)
            n2006 = Equal?(x=w2908, y=10) -> (x = y?=w2904:bool)
            n2007 = case shown="True" w2904 {
              frame False {
              }
              frame True {
                # "password"
                # "password"
                n2008 = local read "Password"() -> (w2921:string)
                n2009 = String To Byte Array(string=w2921) -> (unsigned byte array=w2924:u8[])
                n2010 = String To Byte Array(string="@143$\n") -> (unsigned byte array=w2911:u8[])
                n2011 = Array Size(array=w2924) -> (size(s)=w2920:i32)
                n2012 = Array Size(array=w2911) -> (size(s)=w2916:i32)
                n2013 = for {
                  N: w2920 -> [_]
                  tunnel: w2924 -> [w2937]
                  tunnel: [w2935] -> w2925 mode=indexing
                  tunnel: w2920 -> [w2932]
                  i -> [w2933]
                  n2014 = Decrement(x=w2932) -> (x-1=w2931:i32)
                  n2015 = Index Array(array=w2937, index=w2933) -> (element=w2936:u8)
                  n2016 = Equal?(x=w2933, y=w2931) -> (x = y?=w2930:bool)
                  n2017 = Number To Decimal String(number=w2936) -> (decimal integer string=w2934:string)  [unwired: 1 in]
                  n2018 = Select(t="", s=w2930, f="\r") -> (s? t:f=w2927:string)
                  n2019 = Concatenate Strings(w2934, w2927) -> (w2935:string)
                }
                n2020 = for {
                  N: w2916 -> [_]
                  tunnel: w2911 -> [w2948]
                  tunnel: [w2946] -> w2914 mode=indexing
                  tunnel: w2916 -> [w2943]
                  i -> [w2944]
                  n2021 = Decrement(x=w2943) -> (x-1=w2942:i32)
                  n2022 = Index Array(array=w2948, index=w2944) -> (element=w2947:u8)
                  n2023 = Equal?(x=w2944, y=w2942) -> (x = y?=w2941:bool)
                  n2024 = Number To Decimal String(number=w2947) -> (decimal integer string=w2945:string)  [unwired: 1 in]
                  n2025 = Select(t="", s=w2941, f="\r") -> (s? t:f=w2938:string)
                  n2026 = Concatenate Strings(w2945, w2938) -> (w2946:string)
                }
                n2027 = local read "file path"() -> (w2910:path)
                n2028 = call <vilib>:"Read Characters From File.vi"("file path (dialog if empty)"=w2910) -> ("character string"=w2923:string)  [unwired: 5 in, 3 out]
                "string" <- w2923
                n2029 = flat-sequence {
                  tunnel: [w2926] -> _
                  frame #0 {
                    w2926 = ""
                    n2030 = local write "Password"(w2926) -> ()
                  }
                }
                n2031 = Concatenate Strings(w2914) -> (w2915:string)
                n2032 = Concatenate Strings(w2923) -> (w2922:string)
                n2033 = Concatenate Strings(w2925) -> (w2918:string)
                n2034 = Equal?(x=w2918, y=w2922) -> (x = y?=w2913:bool)
                n2035 = Equal?(x=w2918, y=w2915) -> (x = y?=w2919:bool)
                n2036 = Or(x=w2913, y=w2919) -> (x .or. y?=→"x = y?":bool)
              }
            }
          }
        }
        n2037 = local read "x = y?"() -> (w2894:bool)
        n2038 = And(x="EDIT", y=w2894) -> (x .and. y?=w2892:bool)
        n2039 = case shown="True" w2892 {
          tunnel: [u8 2 ("Disabled") u8 0 ("Disabled")] -> w2891
          tunnel: [w3098 TRUE ("Visible")] -> w2890
          frame False {
            w3098 = FALSE ("Visible")
            n2040 = local write "EDIT 2"(w3098) -> ()
          }
          frame True {
          }
        }
        n2041 = case shown="True" "SAVE" {
          frame False {
          }
          frame True {
            n2042 = stacked-sequence {
              seq-local: [w2953 _ _] -> [_ w3094 _]
              frame #0 {
                w2949 = 0.0 ("number")
                w2950 = 0.0 ("number")
                (unwired) i16 5 ("precision (6)")
                # "[CH1]    - FF\n[CH2]   - TEMPERATURE\n[CH3]    - Humidity\n[CH4]    - AIR TEMP\n[CH5]\\- Visa Uno\n[CH6] \\- Visa Due\n[CH7]  \\- file path\n[CH8]   - Displacement Gain\n[CHA]   - Stroke Gain\n[CHB]   - Stroke PID Gain\n[CHC]   -Language Selection\n[CHD]   -Power +\n[CHE]   -Power_\n[CHF]   -Heater\n[CHG]   -Humidity Wet\n[CHH]   -Humidity Dry\n[CHI]   -Integral Time"
                n2043 = local read "Language Selection"() -> (w2996:enum16{"English", "Russian"})
                n2044 = Path To String(path="File Path") -> (string=w3012:string)
                n2045 = Number To Fractional String(number=w2949, width (-)=i16 10 ("precision (6)"), precision (6)=i16 5) -> (F-format string=w3003:string)  [unwired: 1 in]
                n2046 = Number To Fractional String(number=w2996, width (-)=i16 10 ("precision (6)"), precision (6)=i16 5) -> (F-format string=w2992:string)  [unwired: 1 in]
                n2047 = Number To Fractional String(number=w2950, width (-)=i16 10 ("precision (6)"), precision (6)=i16 5) -> (F-format string=w2986:string)  [unwired: 1 in]
                n2048 = Number To Fractional String(number=w2950, width (-)=i16 10 ("precision (6)"), precision (6)=i16 5) -> (F-format string=w2983:string)  [unwired: 1 in]
                n2049 = Number To Fractional String(number=w2950, width (-)=i16 10 ("precision (6)"), precision (6)=i16 5) -> (F-format string=w2978:string)  [unwired: 1 in]
                n2050 = Number To Fractional String(number=w2950, width (-)=i16 10 ("precision (6)"), precision (6)=i16 5) -> (F-format string=w2975:string)  [unwired: 1 in]
                n2051 = Number To Fractional String(number=w2950, width (-)=i16 10 ("precision (6)"), precision (6)=i16 5) -> (F-format string=w2970:string)  [unwired: 1 in]
                n2052 = local read "Com Port 1"() -> (w2952:refnum<visa-resource-name>)
                n2053 = local read "Com Port 2"() -> (w2951:refnum<visa-resource-name>)
                n2054 = Concatenate Strings(w3012, "\\" ("string")) -> (w3011:string)
                n2055 = Number To Fractional String(number=w2949, width (-)=i16 10 ("precision (6)"), precision (6)=i16 5) -> (F-format string=w3044:string)  [unwired: 1 in]
                n2056 = Number To Fractional String(number=w2949, width (-)=i16 10 ("precision (6)"), precision (6)=i16 5) -> (F-format string=w3043:string)  [unwired: 1 in]
                n2057 = Number To Fractional String(number=w2949, width (-)=i16 10 ("precision (6)"), precision (6)=i16 5) -> (F-format string=w3037:string)  [unwired: 1 in]
                n2058 = Number To Fractional String(number=w2949, width (-)=i16 10 ("precision (6)"), precision (6)=i16 5) -> (F-format string=w3031:string)  [unwired: 1 in]
                n2059 = Number To Fractional String(number=w2949, width (-)=i16 10 ("precision (6)"), precision (6)=i16 5) -> (F-format string=w3004:string)  [unwired: 1 in]
                n2060 = Concatenate Strings("[CHA]" ("string"), w3003, "- Stroke Gain" ("string"), "\r") -> (w2997:string)
                n2061 = Concatenate Strings("[CHC]" ("string"), w2992, "-Language Selection" ("string"), "\r") -> (w2989:string)
                n2062 = Concatenate Strings("[CHD]" ("string"), w2986, "-Power +" ("string"), "\r") -> (w2968:string)
                n2063 = Concatenate Strings("[CHG]" ("string"), w2975, "-Humidity Wet" ("string"), "\r") -> (w2965:string)
                n2064 = Concatenate Strings("[CHH]" ("string"), w2970, "-Humidity Dry" ("string"), "\r") -> (w2964:string)
                n2065 = Concatenate Strings("[CH1]" ("string"), w3044, " - FF" ("string"), "\r") -> (w3042:string)
                n2066 = Concatenate Strings("[CH2]" ("string"), w3043, " - TEMPERATURE" ("string"), "\r") -> (w3041:string)
                n2067 = Concatenate Strings("[CH3]" ("string"), w3037, " - Humidity" ("string"), "\r") -> (w3034:string)
                n2068 = Concatenate Strings("[CH4]" ("string"), w3031, " - AIR TEMP" ("string"), "\r") -> (w3027:string)
                n2069 = Concatenate Strings("[CH5]" ("string"), w2952, "- Visa Uno" ("string"), "\r") -> (w3020:string)
                n2070 = Concatenate Strings("[CH6]" ("string"), w2951, "- Visa Due" ("string"), "\r") -> (w3015:string)
                n2071 = Concatenate Strings("[CH7]" ("string"), w3011, "- file path" ("string"), "\r") -> (w3014:string)
                n2072 = Concatenate Strings("[CH8]" ("string"), w3004, "- Displacement Gain" ("string"), "\r") -> (w3007:string)
                n2073 = Concatenate Strings("[CHE]" ("string"), w2983, "-Power_" ("string"), "\r") -> (w2967:string)
                n2074 = Concatenate Strings("[CHF]" ("string"), w2978, "-Heater" ("string"), "\r") -> (w2966:string)
                n2075 = Concatenate Strings(w3042, w3041, w3034, w3027, w3020, w3015, w3014, w3007, w2997, w2989, w2968, w2967, w2966, w2965, w2964) -> (w2953:string)
                "gain" <- w2953
              }
              frame #1 {
                w3055 = 0.0 ("number")
                n2076 = local read "Camera Port :"() -> (w3058:string)
                n2077 = local read "C3 :"() -> (w3066:refnum<visa-resource-name>)
                n2078 = local read "Com Port 3"() -> (w3067:refnum<visa-resource-name>)
                n2079 = Concatenate Strings("[CH8]" ("string"), w3058, "- Visa Camera" ("string"), "\r") -> (w3057:string)
                n2080 = Concatenate Strings("[CH7]" ("string"), w3066, "- Visa Humidity" ("string"), "\r") -> (w3062:string)
                n2081 = Number To Fractional String(number=w3055, width (-)=i16 10 ("precision (6)"), precision (6)=i16 5) -> (F-format string=w3082:string)  [unwired: 1 in]
                n2082 = Concatenate Strings("[CHL]" ("string"), w3067, "- Visa humid" ("string"), "\r") -> (w3070:string)
                n2083 = Number To Fractional String(number=w3055, width (-)=i16 10 ("precision (6)"), precision (6)=i16 5) -> (F-format string=w3089:string)  [unwired: 1 in]
                n2084 = Concatenate Strings("[CHK]" ("string"), w3082, "-TEMP INTERCEPT" ("string"), "\r") -> (w3078:string)
                n2085 = Concatenate Strings("[SNO]" ("string"), "" ("string"), "-" ("string"), "\r") -> (w3075:string)
                n2086 = Concatenate Strings("[CHJ]" ("string"), w3089, "-AIR TEMP INTERCEPT" ("string"), "\r") -> (w3079:string)
                n2087 = String To Path(string="C:\\LAB-IQ\\calibrate WO 2472.dcf") -> (path=w3068:path)
                n2088 = Concatenate Strings(w3094, w3079, w3078, w3075, w3070, w3062, w3057) -> (w3093:string)
                n2089 = call <vilib>:"Write Characters To File.vi"("append to file? (new file:F)"=FALSE, "character string"=w3093, "file path (dialog if empty)"=w3068) -> ()  [unwired: 2 in, 1 out]
              }
              frame #2 {
                n2090 = local write "Lan flag"(0.0 ("Lan flag")) -> ()
                n2091 = local write "conststatus"(0.0 ("rpm value : 2")) -> ()
                n2092 = local write "SAVE"(FALSE ("OK Button 14")) -> ()
              }
            }
          }
        }
        n2093 = property on="EDIT 2" class="Bool (strict)"("Visible"=w2890) -> ()  [unwired: 2 in, 2 out]
        n2094 = property on="SAVE" class="Bool (strict)"("Visible"=w2890) -> ()  [unwired: 2 in, 2 out]
        n2095 = property on="visa due" class="CmbBox"("Disabled"=w2891) -> ()  [unwired: 2 in, 2 out]
        n2096 = property on="File Path" class="Path"("Disabled"=w2891) -> ()  [unwired: 2 in, 2 out]
        n2097 = property on="Language Selection" class="Enum (strict)"("Visible"=w2890) -> ()  [unwired: 2 in, 2 out]
        n2098 = property on="SPEED OUT:" class="DigNum (strict)"("Disabled"=w2891) -> ()  [unwired: 2 in, 2 out]
      }
    }
    n2099 = local read "RUN"() -> (w2417:bool)
    n2100 = local read "RUN"() -> (w2415:bool)
    n2101 = case shown="True" "EDIT 3" {
      frame False {
      }
      frame True {
        n2102 = local write "EDIT 3"(FALSE ("EDIT 3")) -> ()
        n2103 = local write "Main Tab"(T4."About" ("Main Tab")) -> ()
      }
    }
    n2104 = case shown="False" w2417 {
      frame False {
        n2105 = local read "stopT"() -> (w3105:bool)
        n2106 = case shown="True" w3105 {
          frame False {
          }
          frame True {
            n2107 = local write "stopT"(FALSE) -> ()
          }
        }
      }
      frame True {
        "stopT" <- TRUE
      }
    }
    n2108 = case shown="False" w2415 {
      frame False {
      }
      frame True {
      }
    }
    n2109 = case shown="True" w2407 {
      frame False {
        n2110 = property on="Password 2" class="Str"("Visible"=FALSE) -> ()  [unwired: 2 in, 2 out]
        n2111 = local write "Password 2"("" ("Password")) -> ()
      }
      frame True {
        n2112 = property on="Password 2" class="Str"("Visible"=TRUE) -> ()  [unwired: 2 in, 2 out]
        n2113 = Equal?(x="Password 2", y="HFRR1234") -> (x = y?=w2430:bool)
        n2114 = case shown="True" w2430 {
          tunnel: "Password 2" -> [w2433 _]
          frame False {
            n2115 = String Length(string=w2433) -> (length=w2434:i32)
            n2116 = Greater Than 0?(x=w2434) -> (x > 0?=w2432:bool)
            n2117 = case shown="False" w2432 {
              frame False {
                n2118 = property on="Password 2" class="Str"("Caption.Text"="Password (Advance Setting)") -> ()  [unwired: 2 in, 2 out]
              }
              frame True {
                n2119 = property on="Password 2" class="Str"("Caption.Text"="Incorrect Password!") -> ()  [unwired: 2 in, 2 out]
              }
            }
          }
          frame True {
            n2120 = local write "EDIT 2"(FALSE ("EDIT 2")) -> ()
            n2121 = local write "Password 2"("" ("Password")) -> ()
            n2122 = local write "Main Tab"(T4."Advance" ("Main Tab")) -> ()
            n2123 = local write "Main Dashboard Buttons"(T1."Advance" ("Main Dashboard Buttons")) -> ()
          }
        }
      }
    }
    n2124 = case shown="True" "Prog Uno" {
      frame False {
      }
      frame True {
        n2125 = stacked-sequence {
          frame #0 {
            n2126 = Delete(path (use dialog)=path "C:/LAB-IQ-NXT/UNOCOMPILE.bat" ("working directory")) -> ()  [unwired: 4 in, 3 out]
          }
          frame #1 {
            n2127 = local read "Com Port 1"() -> (w2872:refnum<visa-resource-name>)
            n2128 = Concatenate Strings("cmd.exe /c \"mode " ("command line"), w2872, ":1200,n,8,1\"\n" ("command line")) -> (w2877:string)
            n2129 = Concatenate Strings(w2877, "CD\\\nCD WinDucom\navrdude -C avrdude.conf -v -patmega328p -carduino -P" ("command line"), w2872, " -b115200 -D -Uflash:w:UNO_V20.hex:i\n" ("command line"), "\r") -> (w2879:string)
            "STR" <- w2879
            n2130 = call <vilib>:"Write Characters To File.vi"("append to file? (new file:F)"=FALSE, "character string"=w2879, "file path (dialog if empty)"=path "C:/LAB-IQ/UNOCOMPILE.bat" ("working directory")) -> ()  [unwired: 2 in, 1 out]
          }
          frame #2 {
            n2131 = disable-structure shown="Disabled" {
              frame Disabled {
                w2883 = "cmd.exe  /c \"C:\\LAB-IQ-NXT\\UNOCOMPILE.bat\"" ("string")
                n2132 = local write "Prog Uno"(FALSE ("run minimized? (F)")) -> ()
                n2133 = call <vilib>:"System Exec.vi"("expected output size  (4096)"=u32 65535, "run minimized? (F)"=FALSE, "wait until completion? (T)"=TRUE ("run minimized? (F)"), "working directory"=path "C:/LAB-IQ-NXT", "standard input"=w2883, "command line"=w2883) -> ("error out"=w2882:errorcluster, "standard output"=→"String 42":string)  [unwired: 2 in, 2 out]
                "error out 3" <- w2882
                n2134 = flat-sequence {
                  tunnel: w2882 -> [_]
                  frame #0 {
                  }
                }
              }
              frame Enabled {
              }
            }
          }
        }
      }
    }
    n2135 = case shown="\"ISO 12156\"" "TEST STANDARD" {
      frame "ASTM D6079", Default {
        w2852 = 50.0 ("Hz")
        w2853 = 53.0 ("Set Rh")
        w2855 = 1.0 ("Set Strk")
        w2854 = 60.0 ("Set Temp")
        # "astm hide"
        n2136 = local write "NORMAL LOAD"(200.0 ("NORMAL LOAD")) -> ()
        n2137 = local write "Set Strk"(w2855) -> ()
        n2138 = local write "Set Hz"(w2852) -> ()
        n2139 = local write "Set Temp"(w2854) -> ()
        n2140 = local write "Set Rh"(w2853) -> ()
        n2141 = local write "test time"(75.0 ("test time")) -> ()
        n2142 = local write "Set Stroke:"(w2855) -> ()
        n2143 = local write "Set Humidity:"(w2853) -> ()
        n2144 = local write "Set Frequency:"(w2852) -> ()
        n2145 = local write "Set Temperature:"(w2854) -> ()
        "Test Standard" <- "ASTM D6079" ("Test Standard 2")
      }
      frame "ISO 12156" {
        n2146 = local write "Set Strk"(1.0 ("Set Strk")) -> ()
        n2147 = local write "NORMAL LOAD"(200.0 ("NORMAL LOAD")) -> ()
        n2148 = local write "Set Temp"(60.0 ("Set Temp")) -> ()
        n2149 = local write "test time"(75.0 ("test time")) -> ()
        n2150 = local write "Set Hz"(50.0 ("Hz")) -> ()
        n2151 = local write "Set Rh"(53.0 ("Set Rh")) -> ()
      }
      frame "CEC F-096-A-06" {
        n2152 = local write "Set Strk"(1.0 ("Set Strk")) -> ()
        n2153 = local write "NORMAL LOAD"(200.0 ("NORMAL LOAD")) -> ()
        n2154 = local write "Set Temp"(60.0 ("Set Temp")) -> ()
        n2155 = local write "test time"(75.0 ("test time")) -> ()
        n2156 = local write "Set Hz"(50.0 ("Hz")) -> ()
        n2157 = local write "Set Rh"(53.0 ("Set Rh")) -> ()
      }
